vi "Number To Boolean.vi"(1 "Number":u32) -> (0 "Boolean Value":bool)   [LabVIEW 2012]
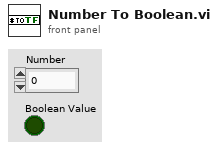
[diagram p1: front panel]
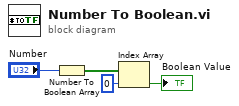
[diagram p0: block diagram]
diagram:
  n1 = Number To Boolean Array(number="Number") -> (Boolean array=w4:bool[])
  n2 = Index Array(array=w4, index=0) -> (element=→"Boolean Value":bool)
